vi "GetCopyExactDependencies.vi"(8 "Error In":errorcluster, 10 "Package Version":string, 11 "Package Name":string) -> (0 "Error Out":errorcluster, 3 "Copy Exact Dependencies":string[](array[string]))   [LabVIEW 2019, in "CEPM.lvlib"]
uses:
  CEPM.lvlib
  <vilib>/National Instruments/NIPM API (Beta)/NIPM_API.lvlib
panel:
  out "Same?":bool
  out "Same?":bool[](array[boolean])
  out "Array":string[](array[string])
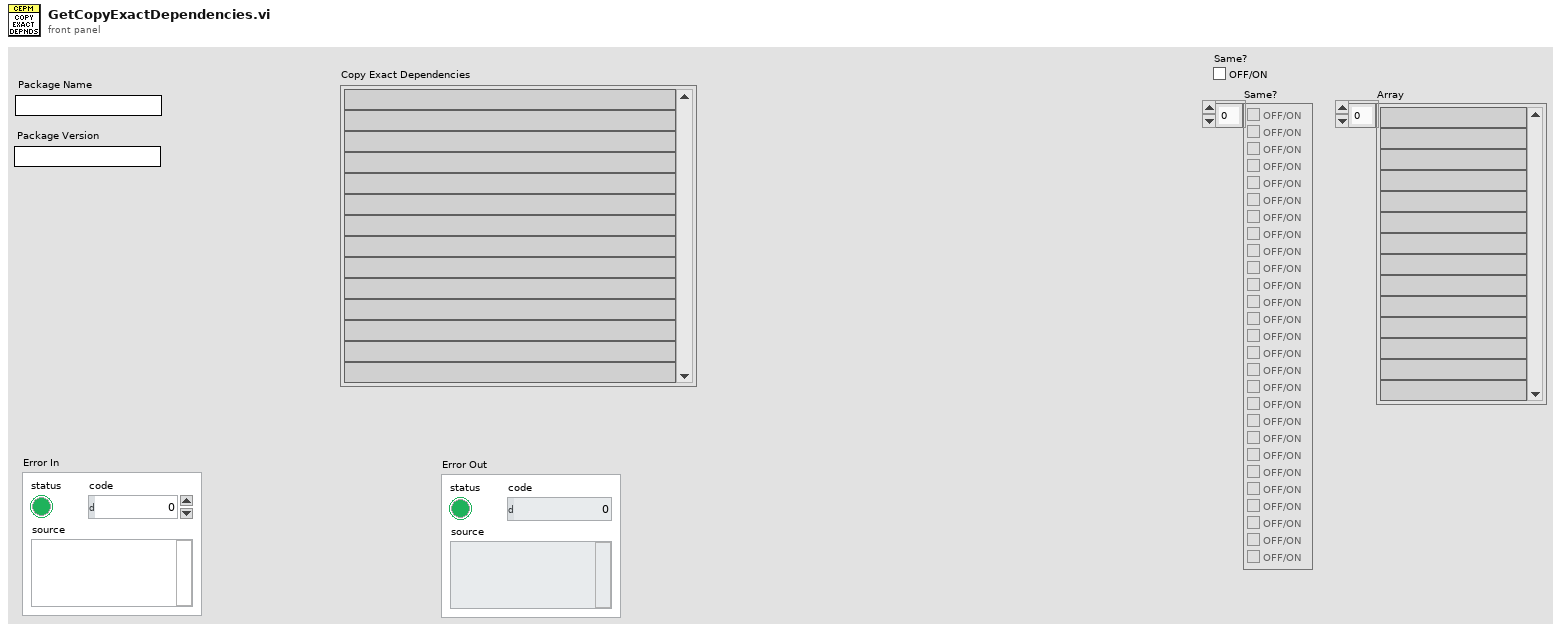
[diagram p1: front panel]
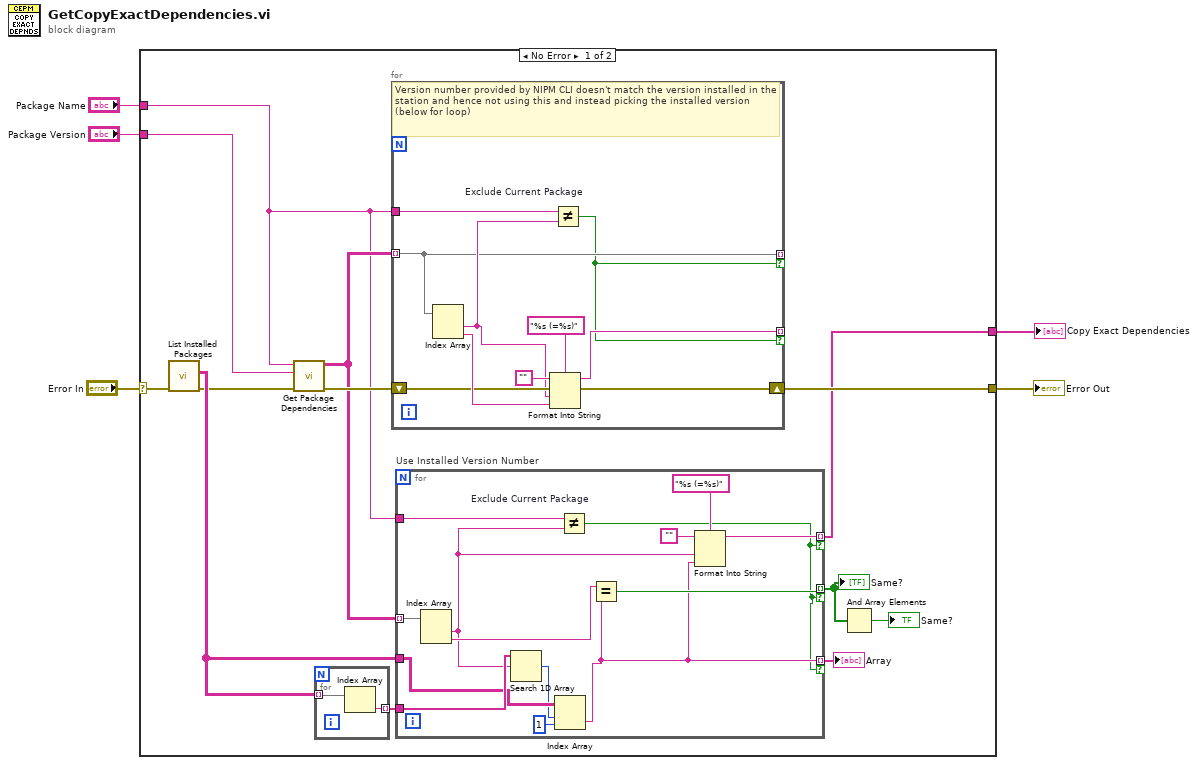
[diagram p0: block diagram]
diagram:
  n1 = case shown="No Error" "Error In" {
    selector: "Error In" -> [w7 w45]
    tunnel: "Package Version" -> [w18 _]
    tunnel: [w16 w45] -> w3
    tunnel: "Package Name" -> [w9 _]
    tunnel: [w8 _] -> w1
    frame No Error {
      n2 = call <vilib>:"List Installed Packages.vi"("error in"=w7) -> ("error out"=w6:errorcluster, "installed packages"=w13:string[][])  [unwired: 9 in]
      n3 = call <vilib>:"Get Package Dependencies.vi"("error in"=w6, "version"=w18, "package name"=w9) -> ("error out"=w17:errorcluster, "package dependencies"=w15:string[][])  [unwired: 7 in]
      n4 = for {
        tunnel: w13 -> [w20] mode=indexing
        tunnel: [w19] -> w14 mode=indexing
        n5 = Index Array(array=w20) -> (element=w19:string)  [unwired: 1 in]
      }
      n6 = for {
        tunnel: w15 -> [w36] mode=indexing
        tunnel: [w41] -> _ mode=indexing if=w35
        shift-right: [w39] -> w16
        shift-left: w17 -> [w40]
        tunnel: w9 -> [w37]
        tunnel: [w36] -> _ mode=indexing if=w35
        # "Version number provided by NIPM CLI doesn't match the version installed in the station and hence not using this and instead picking the installed version (below for loop)"
        n7 = Index Array(array=w36) -> (element #1=w38:string, element #2=w42:string)  [unwired: 2 in]
        n8 = Format Into String(format string="%s (=%s)", initial string="", error in=w40, w38, w42) -> (resulting string=w41:string, error out=w39:errorcluster)
        n9 = Not Equal? "Exclude Current Package"(x=w37, y=w38) -> (x != y?=w35:bool)
      }
      n10 = for "Use Installed Version Number" {
        tunnel: w15 -> [w34] mode=indexing
        tunnel: w14 -> [w33]
        tunnel: w13 -> [w32]
        tunnel: [w23] -> w12 mode=indexing if=w21
        tunnel: [w28] -> w11 mode=indexing if=w21
        tunnel: w9 -> [w27]
        tunnel: [w22] -> w8 mode=indexing if=w21
        n11 = Index Array(array=w34) -> (element #1=w24:string, element #2=w29:string)  [unwired: 2 in]
        n12 = Search 1D Array(1D array=w33, element=w24) -> (index of element=w31:i32)  [unwired: 1 in]
        n13 = Index Array(array=w32, index (row)=w31, index (col)=1 ("disabled index (col)")) -> (element=w23:string)
        n14 = Not Equal? "Exclude Current Package"(x=w27, y=w24) -> (x != y?=w21:bool)
        n15 = Equal?(x=w29, y=w23) -> (x = y?=w28:bool)
        n16 = Format Into String(format string="%s (=%s)", initial string="", w24, w23) -> (resulting string=w22:string)  [unwired: 1 in, 1 out]
      }
      "Array" <- w12
      "Same?" <- w11
      n17 = And Array Elements(Boolean array=w11) -> (logical AND=→"Same?":bool)
    }
    frame Error {
    }
  }
  "Error Out" <- w3
  "Copy Exact Dependencies" <- w1
